vi "GetActualSteerAngles.vi"(10 "Zero Relative Encoder":bool, 11 "Relative Encoders?":bool) -> (3 "Robot Motion Commands":T1)   [LabVIEW 2018]
doc: "Input: \nName: Relative Encoders? Type: Boolean Default: F (F=absolute, T=relative)\nName: Zero Relative Encoder Type: Boolean Default: F\n\nOutput: \nName: Actual Angles Type: Robot Pivot Motion Commands\n\nPurpose: \nTo get the actual angles from the encoders in units of degrees and align the neutral angle orientation with the frame on the robot\n\nAlgorithm: \nGet the steer angle encoder objects using the corresponding names found in the begin function. Different objects and functions will be needed if relative or absolute encoders are used. \n\nIf Relative Encoders input is False, get the absolute encoder objects and use the appropriate functions to read the encoder channels and convert to angle in degrees. Values should be between -180 and +180. Hard coded offsets should be used to align the motors with the frame and set that particular rotation as 0 degrees. Each encoder will require a different offset value. Bundle values into appropriate ‘Steer Angle (deg)’ in the Robot Pivot Motion Commands cluster.\n\nIf Relative Encoders input is True, get the relative encoder objects and use the appropriate functions to read the encoder channels and convert to angle in degrees. Values should be between -180 and +180. Bundle values into appropriate ‘Steer Angle (deg)’ in the Robot Pivot Motion Commands cluster.\n\nIf the Zero Relative Encoder input is True then get the relative encoder objects and use the appropriate functions to Reset all encoder channels."
uses:
  Robot Pivot Motion Commands.ctl
  Pivot Motor Commands.ctl
  Robot Drive Mode.ctl
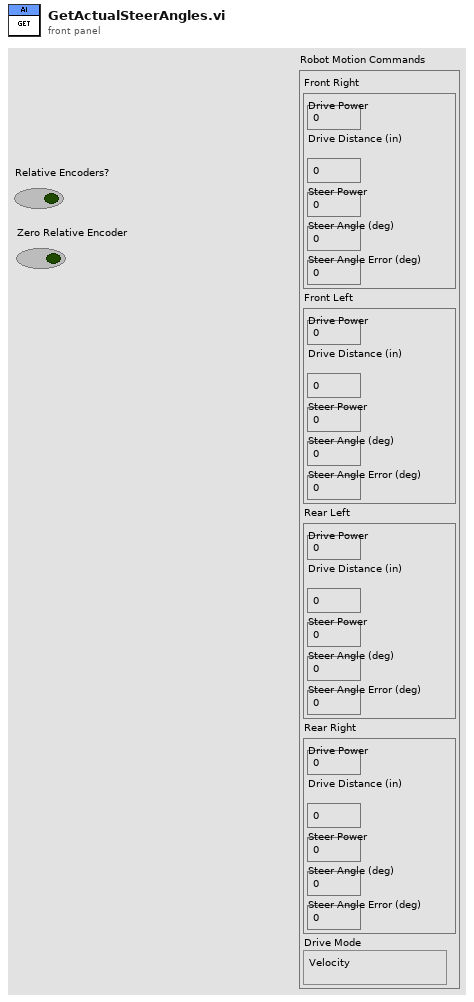
[diagram p1: front panel]
types:
  T1 = typedef "Robot Pivot Motion Commands.ctl" = cluster{"Front Right":T2, "Front Left":T2, "Rear Left":T2, "Rear Right":T2, "Drive Mode":T3}
  T2 = typedef "Pivot Motor Commands.ctl" = cluster{"Drive Power":dbl, "Drive Distance (in)":dbl, "Steer Power":dbl, "Steer Angle (deg)":dbl, "Steer Angle Error (deg)":dbl}
  T3 = typedef "Robot Drive Mode.ctl" = enum16{"Velocity", "Distance"}
  T4 = typedef "WPI_AnalogChannelDevRef.ctl" = cluster{"DevStatus":errorcluster, "Analog Channel":T5}
  T5 = typedef "FPGA_AIChannel.ctl" = enum8{"AI 0", "AI 1", "AI 2", "AI 3", "AI MXP 0", "AI MXP 1", "AI MXP 2", "AI MXP 3", "Invalid"}
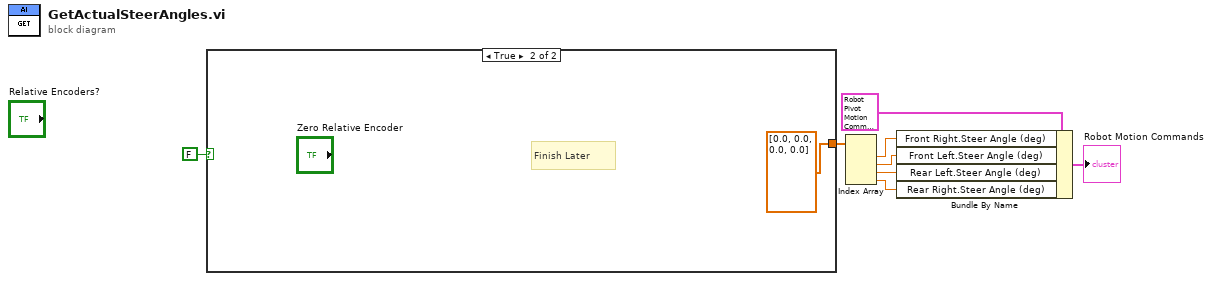
[diagram p0: block diagram]
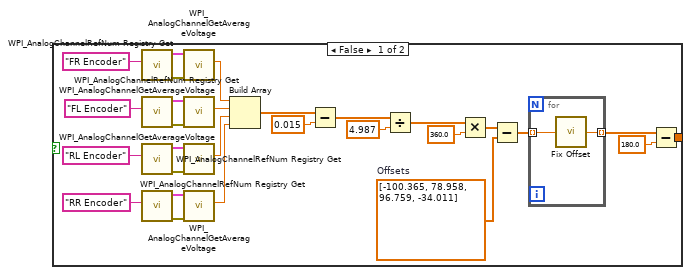
[diagram p2: hidden frame]
diagram:
  n1 = case shown="True" FALSE {
    tunnel: [w9 dbl[] [0.0, 0.0, 0.0, 0.0]] -> w6
    frame False {
      w12 = dbl[] [-100.365, 78.958, 96.759, -34.011]  # Offsets
      n2 = call <vilib>:"WPI_AnalogChannelRefNum Registry Get.vi"("refnum name"="FR Encoder") -> ("error out"=w36:errorcluster, "AIDeviceRef"=w35:T4)  [unwired: 9 in]
      n3 = call <vilib>:"WPI_AnalogChannelRefNum Registry Get.vi"("refnum name"="FL Encoder") -> ("error out"=w33:errorcluster, "AIDeviceRef"=w32:T4)  [unwired: 9 in]
      n4 = call <vilib>:"WPI_AnalogChannelRefNum Registry Get.vi"("refnum name"="RL Encoder") -> ("error out"=w30:errorcluster, "AIDeviceRef"=w29:T4)  [unwired: 9 in]
      n5 = call <vilib>:"WPI_AnalogChannelRefNum Registry Get.vi"("refnum name"="RR Encoder") -> ("error out"=w27:errorcluster, "AIDeviceRef"=w26:T4)  [unwired: 9 in]
      n6 = call <vilib>:"WPI_AnalogChannelGetAverageVoltage.vi"("error in (no error)"=w36, "AIDeviceRef"=w35) -> ("Voltage"=w17:dbl)  [unwired: 7 in, 2 out]
      n7 = call <vilib>:"WPI_AnalogChannelGetAverageVoltage.vi"("error in (no error)"=w33, "AIDeviceRef"=w32) -> ("Voltage"=w16:dbl)  [unwired: 7 in, 2 out]
      n8 = call <vilib>:"WPI_AnalogChannelGetAverageVoltage.vi"("error in (no error)"=w30, "AIDeviceRef"=w29) -> ("Voltage"=w15:dbl)  [unwired: 7 in, 2 out]
      n9 = call <vilib>:"WPI_AnalogChannelGetAverageVoltage.vi"("error in (no error)"=w27, "AIDeviceRef"=w26) -> ("Voltage"=w14:dbl)  [unwired: 7 in, 2 out]
      n10 = Build Array(w17, w16, w15, w14) -> (w13:dbl[])
      n11 = Subtract(x=w13, y=0.015) -> (x-y=w23:dbl[])
      n12 = Divide(x=w23, y=4.987) -> (x/y=w21:dbl[])
      n13 = Multiply(x=w21, y=360.0) -> (x*y=w19:dbl[])
      n14 = Subtract(x=w19, y=w12) -> (x-y=w11:dbl[])
      n15 = for {
        tunnel: w11 -> [w38] mode=indexing
        tunnel: [w37] -> w10 mode=indexing
        n16 = call "Fix Offset.vi"("Input Angle"=w38) -> ("Output Angle"=w37:dbl)
      }
      n17 = Subtract(x=w10, y=180.0) -> (x-y=w9:dbl[])
    }
    frame True {
      # "Finish Later"
    }
  }
  n18 = Index Array(array=w6) -> (element #1=w5:dbl, element #2=w4:dbl, element #3=w3:dbl, element #4=w2:dbl)  [unwired: 4 in]
  n19 = Bundle By Name(cluster=T1 {"Front Right"={"Drive Power"=0.0, "Drive Distance (in)"=0.0, "Steer Power"=0.0, "Steer Angle (deg)"=0.0, "Steer Angle Error (deg)"=0.0}, "Front Left"={"Drive Power"=0.0, "Drive Distance (in)"=0.0, "Steer Power"=0.0, "Steer Angle (deg)"=0.0, "Steer Angle Error (deg)"=0.0}, "Rear Left"={"Drive Power"=0.0, "Drive Distance (in)"=0.0, "Steer Power"=0.0, "Steer Angle (deg)"=0.0, "Steer Angle Error (deg)"=0.0}, "Rear Right"={"Drive Power"=0.0, "Drive Distance (in)"=0.0, "Steer Power"=0.0, "Steer Angle (deg)"=0.0, "Steer Angle Error (deg)"=0.0}, "Drive Mode"=enum."Velocity"} ("Robot Motion Commands"), "Front Right.Steer Angle (deg)"=w5, "Front Left.Steer Angle (deg)"=w4, "Rear Left.Steer Angle (deg)"=w3, "Rear Right.Steer Angle (deg)"=w2) -> (→"Robot Motion Commands":T1)
